vi "MolarityCalc.vi"() -> ()   [LabVIEW 2015]
panel:
  out "Total Mass\nfrom Molar ratio":dbl
  out "Volume of Solvent needed (ml)":dbl
  in  "Weight Percent":T1
  out "Solute Volume (ml)":dbl
  in  "Liquid Molarity":T2
  in  "Solid\nMolar Ratio":T3
  out "Total Moles":dbl
  in  "stop":bool
  out "Mass of Chemical 2":dbl
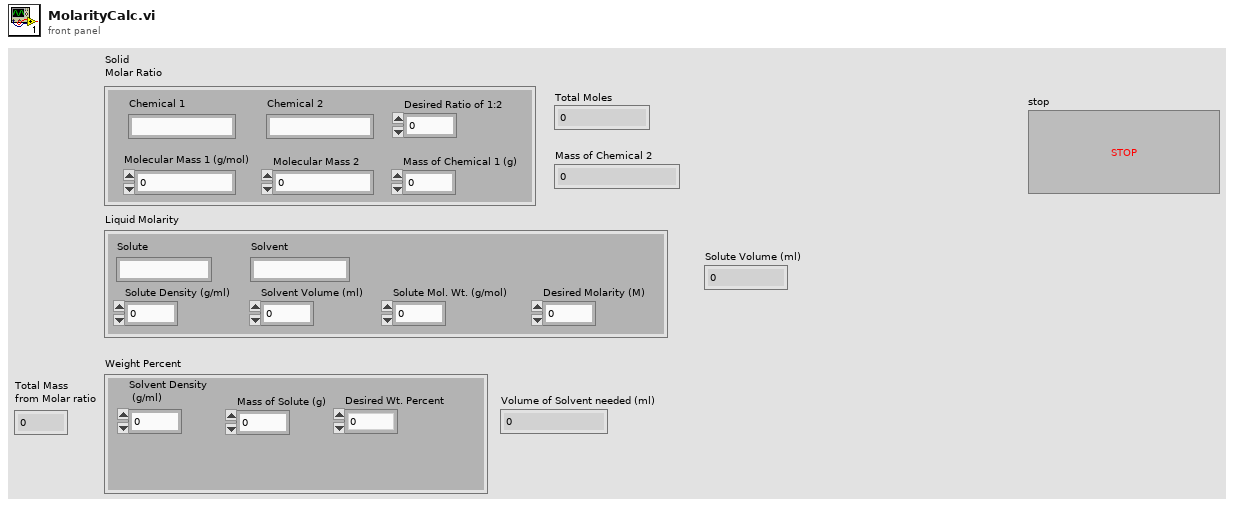
[diagram p1: front panel]
types:
  T1 = cluster{"Solvent Density\n (g/ml)":dbl, "Mass of Solute (g)":dbl, "Desired Wt. Percent":dbl}
  T2 = cluster{"Solute":string, "Solvent":string, "Solute Density (g/ml)":dbl, "Solvent Volume (ml)":dbl, "Desired Molarity (M)":dbl, "Solute Mol. Wt. (g/mol)":dbl}
  T3 = cluster{"Molecular Mass 2":dbl, "Chemical 2":string, "Molecular Mass 1 (g/mol)":dbl, "Chemical 1":string, "Desired Ratio of 1:2":dbl, "Mass of Chemical 1 (g)":dbl}
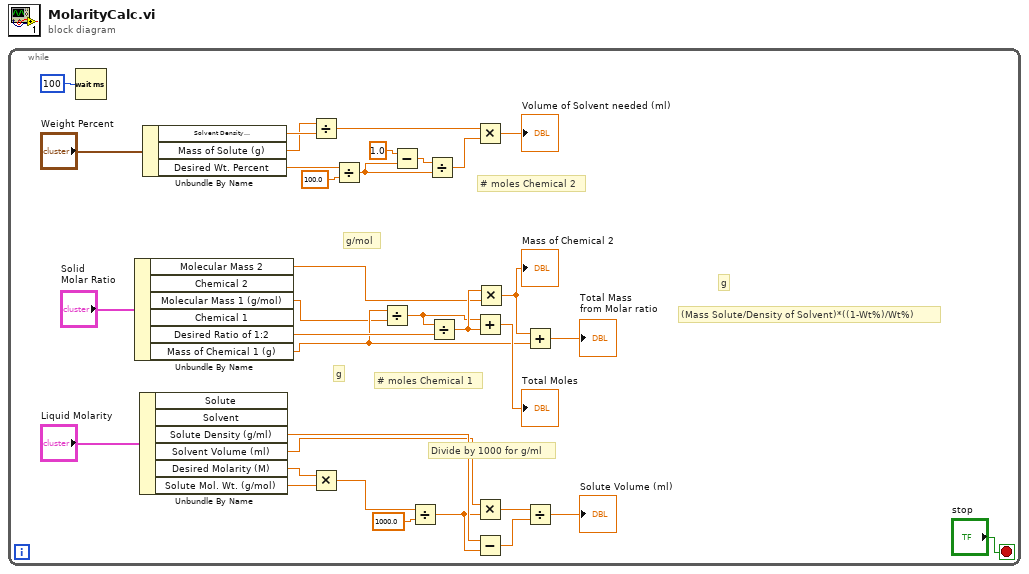
[diagram p0: block diagram]
diagram:
  n1 = while {
    stop <- "stop" stop-if-true
    # "(Mass Solute/Density of Solvent)*((1-Wt%)/Wt%)"
    # "Divide by 1000 for g/ml"
    # "g"
    # "# moles Chemical 2"
    # "# moles Chemical 1"
    # "g"
    # "g/mol"
    n2 = Wait (ms)(milliseconds to wait=u32 100) -> ()  [unwired: 1 out]
    n3 = Unbundle By Name("Solid\nMolar Ratio") -> ("Molecular Mass 2"=w2:dbl, "Molecular Mass 1 (g/mol)"=w1:dbl, "Desired Ratio of 1:2"=w28:dbl, "Mass of Chemical 1 (g)"=w5:dbl)  [unwired: 2 out]
    n4 = Unbundle By Name("Liquid Molarity") -> ("Solute Density (g/ml)"=w22:dbl, "Solvent Volume (ml)"=w19:dbl, "Desired Molarity (M)"=w25:dbl, "Solute Mol. Wt. (g/mol)"=w26:dbl)  [unwired: 2 out]
    n5 = Unbundle By Name("Weight Percent") -> ("Solvent Density\n (g/ml)"=w13:dbl, "Mass of Solute (g)"=w12:dbl, "Desired Wt. Percent"=w8:dbl)
    n6 = Divide(x=w12, y=w13) -> (x/y=w10:dbl)
    n7 = Multiply(x=w25, y=w26) -> (x*y=w24:dbl)
    n8 = Divide(x=w8, y=100.0) -> (x/y=w6:dbl)
    n9 = Divide(x=w5, y=w1) -> (x/y=w31:dbl)
    n10 = Subtract(x=1.0, y=w6) -> (x-y=w14:dbl)
    n11 = Divide(x=w24, y=1000.0) -> (x/y=w21:dbl)
    n12 = Divide(x=w14, y=w6) -> (x/y=w11:dbl)
    n13 = Divide(x=w31, y=w28) -> (x/y=w32:dbl)
    n14 = Multiply(x=w10, y=w11) -> (x*y=→"Volume of Solvent needed (ml)":dbl)
    n15 = Add(x=w31, y=w32) -> (x+y=→"Total Moles":dbl)
    n16 = Multiply(x=w19, y=w21) -> (x*y=w18:dbl)
    n17 = Subtract(x=w22, y=w21) -> (x-y=w20:dbl)
    n18 = Multiply(x=w32, y=w2) -> (x*y=w4:dbl)
    "Mass of Chemical 2" <- w4
    n19 = Add(x=w4, y=w5) -> (x+y=→"Total Mass\nfrom Molar ratio":dbl)
    n20 = Divide(x=w18, y=w20) -> (x/y=→"Solute Volume (ml)":dbl)
  }
